vi "Set Output Switch Direction.vi"(8 "error in (no error)":errorcluster, 10 "After delay":bool, 11 "RP Instrument in":refnum<class "RP Instrument.lvclass">) -> (0 "error out":errorcluster, 3 "RP Instrument out":refnum<class "RP Instrument.lvclass">)   [LabVIEW 2024, in "RP Instrument.lvclass"]
uses:
  RP Instrument.lvclass
  RP Command.ctl
  RP Instrument.lvclass/RP Instrument.ctl
  RP Communicator/RP Communicator.lvclass
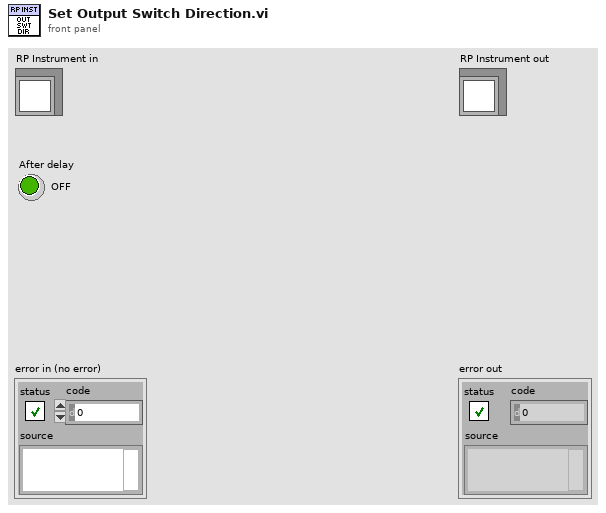
[diagram p1: front panel]
types:
  T1 = typedef "RP Command.ctl" = enum16{"Reset", "Read IDN", "Stop server", "Get status", "Get temperature", "Connect client", "Arm", "Software trigger", "Get whole buffer", "Get chunk", "System call", "Get config", "Set config", "Recieve data", "Recieve Calibartion", "Transmit data"}
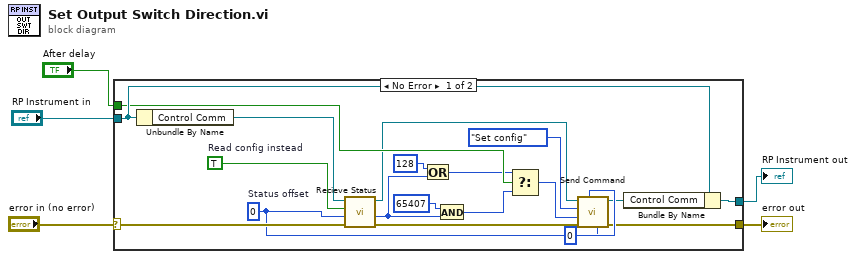
[diagram p0: block diagram]
diagram:
  n1 = case shown="No Error" "error in (no error)" {
    selector: "error in (no error)" -> [w21 w26]
    tunnel: [w9 w26] -> w4
    tunnel: [w8 w25] -> w2
    tunnel: "RP Instrument in" -> [w24 w25]
    tunnel: "After delay" -> [w20 _]
    frame No Error {
      w12 = u64 0  # Status offset
      w22 = TRUE  # Read config instead
      n2 = Unbundle By Name(w24) -> ("Control Comm"=w23:refnum<class "RP Communicator.lvclass">)
      n3 = call-dynamic "Recieve Status.vi"("error in (no error)"=w21, "Status offset"=w12, "Read config instead"=w22, "RP Communicator in"=w23) -> ("error out"=w10:errorcluster, "Status response"=w16:u32, "RP Communicator out"=w14:refnum<class "RP Communicator.lvclass">)  [unwired: 5 in]
      n4 = Or(x=u32 128, y=w16) -> (x .or. y?=w15:u32)
      n5 = And(x=u32 65407, y=w16) -> (x .and. y?=w18:u32)
      n6 = Select(t=w15, s=w20, f=w18) -> (s? t:f=w11:u32)
      n7 = call-dynamic "Send Command.vi"("bytes to read"=0, "Config offset"=w12, "error in (no error)"=w10, "Command payload"=w11, "Command number"=RP_Command."Set config", "RP Communicator in"=w14) -> ("error out"=w9:errorcluster, "RP Communicator out"=w7:refnum<class "RP Communicator.lvclass">)  [unwired: 3 in, 1 out]
      n8 = Bundle By Name(cluster=w24, "Control Comm"=w7) -> (w8:refnum<class "RP Instrument.lvclass">)
    }
    frame Error {
    }
  }
  "error out" <- w4
  "RP Instrument out" <- w2
